vi "SA40144D.20210624 1D only.vi"() -> ()   [LabVIEW 2020]
uses:
  <vilib>/Analysis/baseanly.llb/Mean (DBL).vi
  <userlib>/_OpenG.lib/file/file.llb/Build Path - Traditional__ogtk.vi
  <userlib>/LevyLab/LV to ITX/Data/Data.lvclass
  <userlib>/LevyLab/XY Utilities/xy_utilities.lvlib
  <vilib>/Analysis/NI_AALBase.lvlib
panel:
  in  "Temps to keep (Lifespan)":i32=26
  out "Lifespan vs Temp (hrs)":cluster{i32[], dbl[]}[](graph)
  out "E_a":dbl[](array[numeric])
  out "Arrhenius":T1(graph)
  in  "Temps to keep (Arrhenius fit)":i32=26
  out "G2T vs t":T1(graph)
  out "G4T vs t":T1(graph)
  out "X5 - I-":T1(graph)
  out "X6 - dV":T1(graph)
  out "Temp vs t":T1(graph)
  out "G2T BG vs t":T1(graph)
  in  "Source Voltage":dbl=0.1
  in  "Init Temp":i32=275
  in  "Temp Step":i32=5
  in  "Final Temp":i32=360
  in  "Data File":path=path "G:/My Drive/ansom/Data/PPMS 2/SA40144D.20210624/00 - 1D only/SA40144D.20210624.000000.dat"
  in  "Trimming":i32=400
  in  "Update":bool
  in  "OK":bool
  out "error out":errorcluster
  in  "error in (no error)":errorcluster
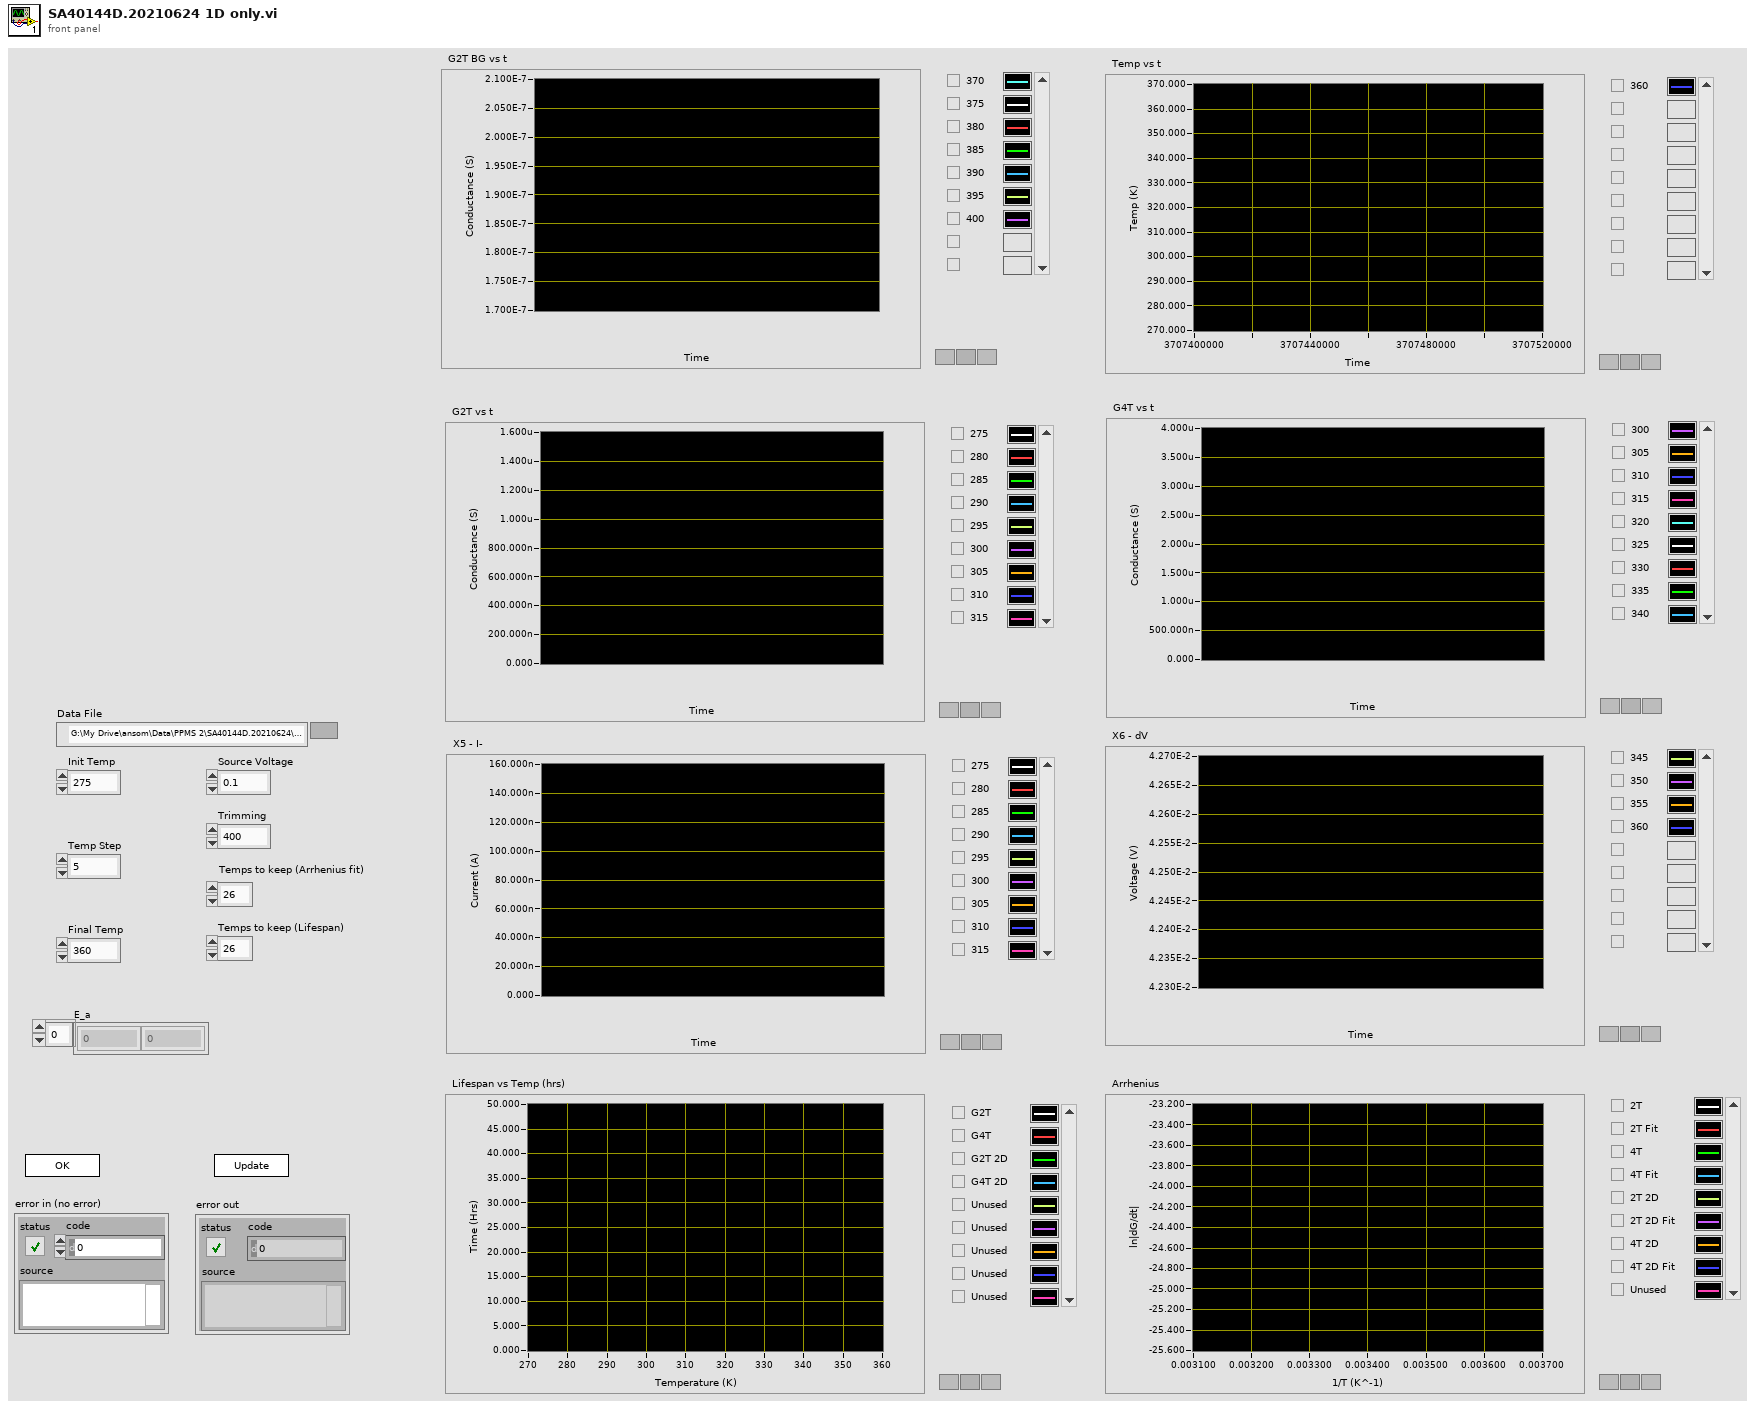
[diagram p1: front panel]
types:
  T1 = cluster{"Data":dbl[], "Best Exponential Fit":dbl[]}[]
  T2 = enum32{"Invalid", "Standard", "Closed", "Hidden", "Minimized", "Maximized"}
  T3 = enum32{"invalid app kind", "Development System", "Run Time System", "Student Edition", "Embedded LabVIEW", "Evaluation", "Custom"}
  T4 = cluster{"Core":cluster{"Current VI Reference":refnum<vi>, "Close Panel on Exit?":bool}, "G2T 1D":cluster{dbl[], dbl[]}[], "G4T 1D":cluster{dbl[], dbl[]}[], "X11":cluster{dbl[], dbl[]}[], "X15":cluster{dbl[], dbl[]}[], "Temp":cluster{dbl[], dbl[]}[], "G2T BG":cluster{dbl[], dbl[]}[], "Source Voltage":dbl, "Final Temp":i32, "Init Temp":i32, "Temp Step":i32, "Data File":path, "Trimming":i32}
  T5 = cluster{"Current VI Reference":refnum<vi>, "Close Panel on Exit?":bool}
  T6 = typedef "Data.lvclass/Dictionary--cluster.ctl" = cluster{"key":string, "value":variant}
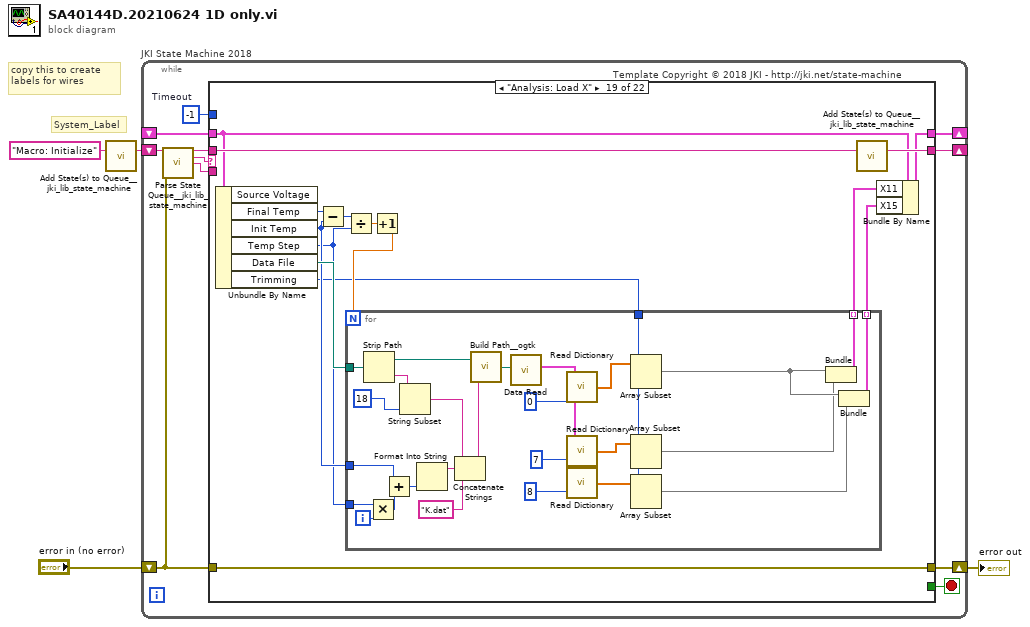
[diagram p0: block diagram]
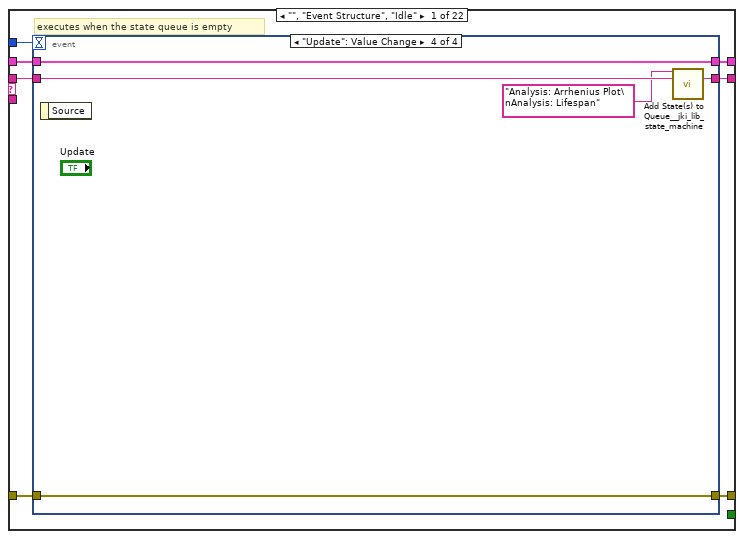
[diagram p2: hidden frame]
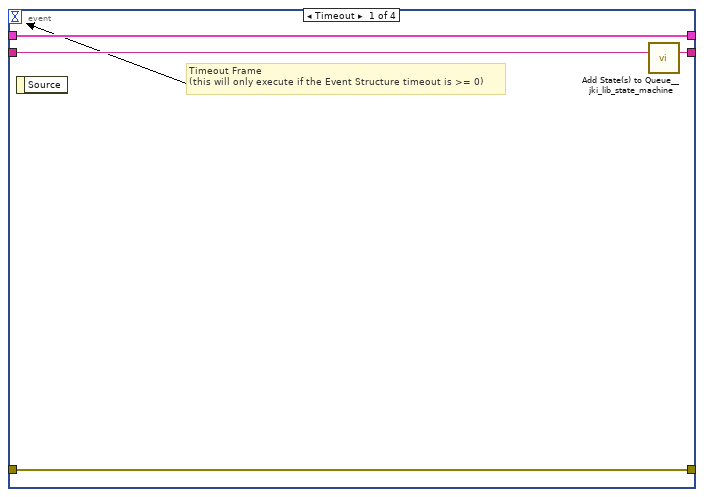
[diagram p3: hidden frame]
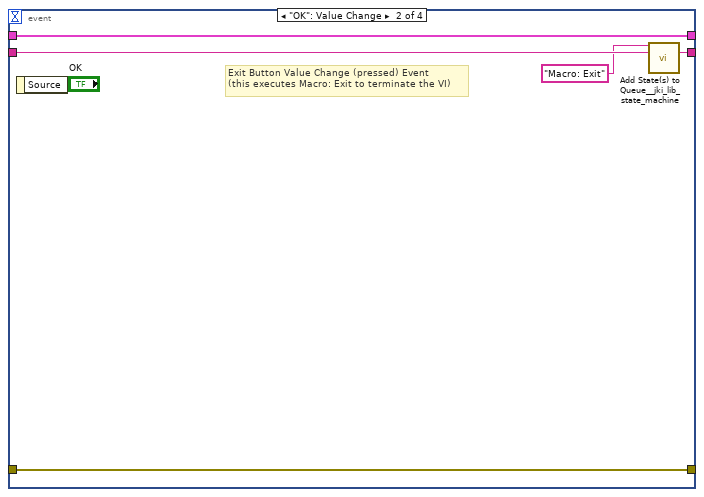
[diagram p4: hidden frame]
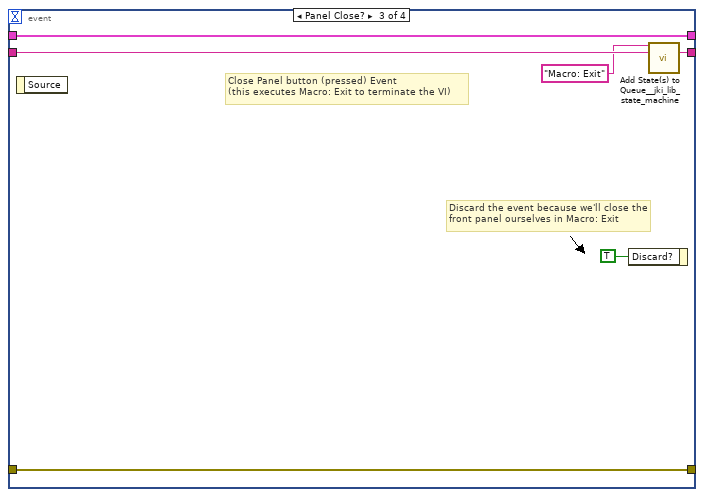
[diagram p5: hidden frame]
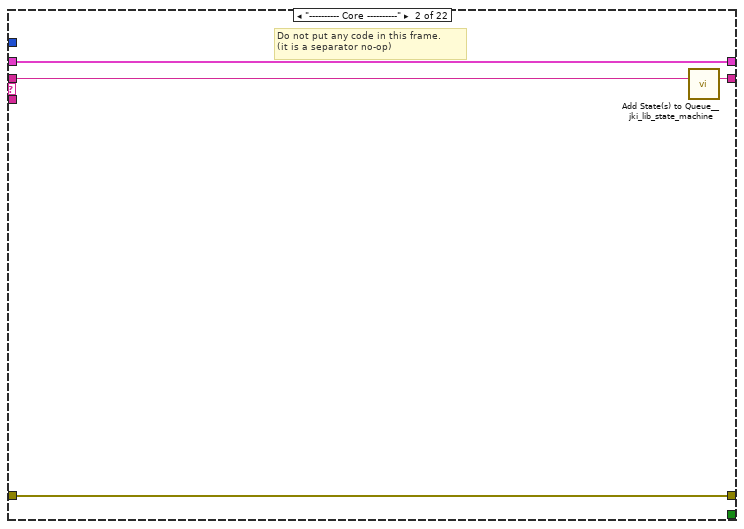
[diagram p6: hidden frame]
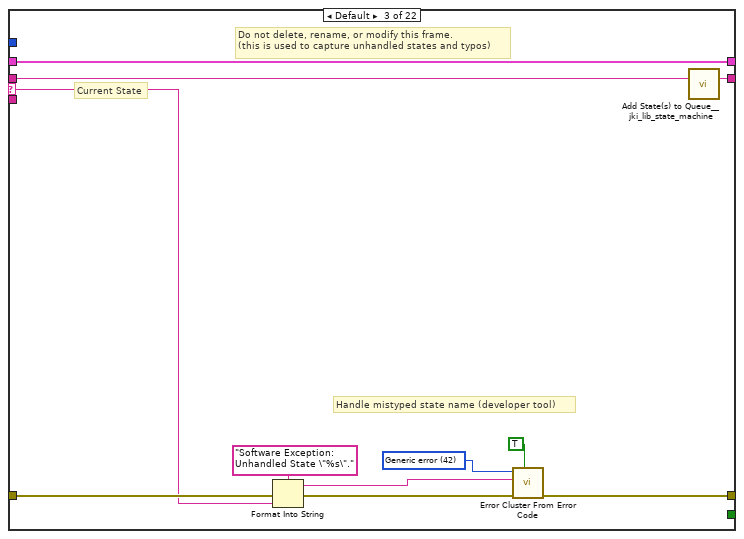
[diagram p7: hidden frame]
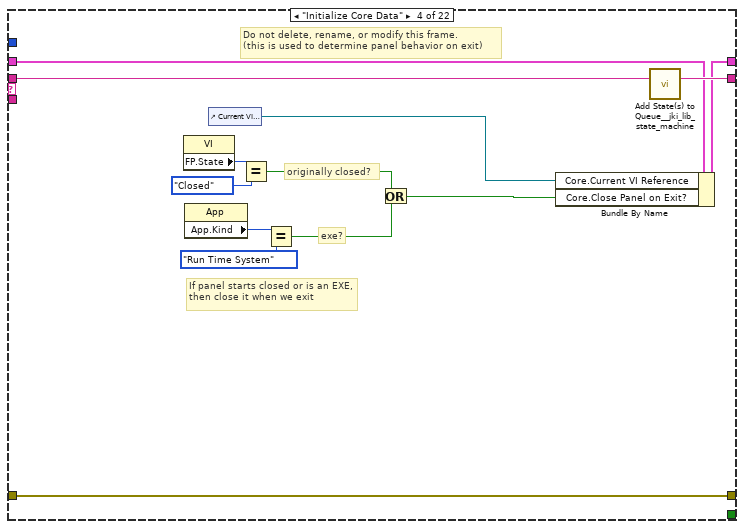
[diagram p8: hidden frame]
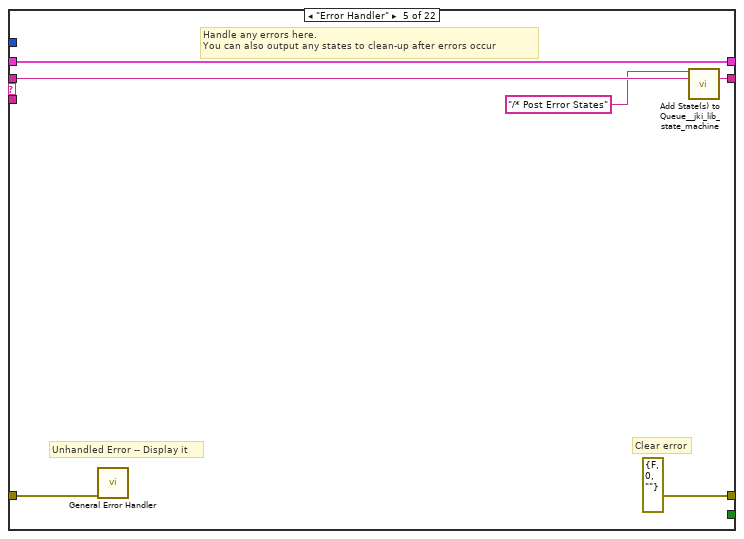
[diagram p9: hidden frame]
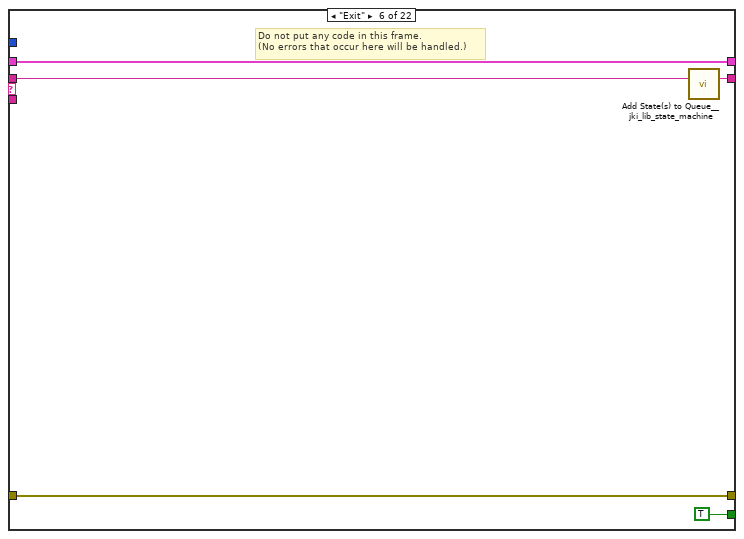
[diagram p10: hidden frame]
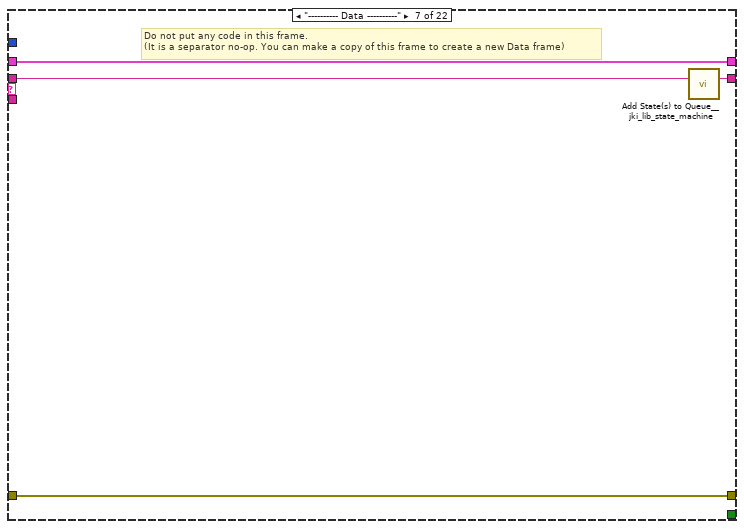
[diagram p11: hidden frame]
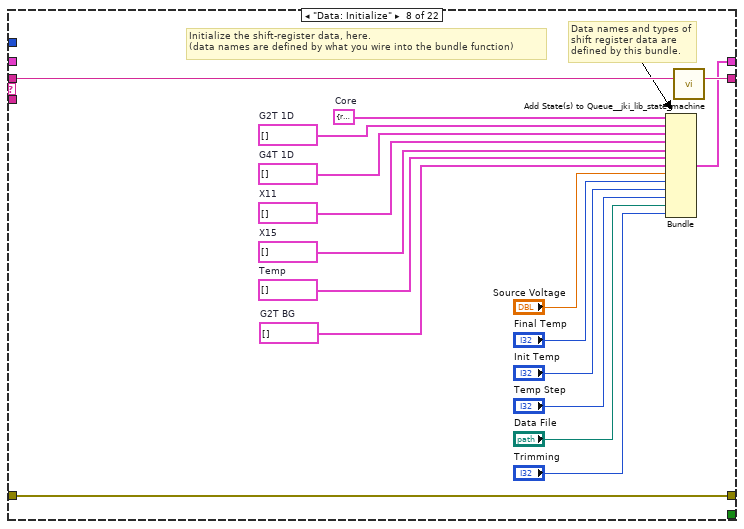
[diagram p12: hidden frame]
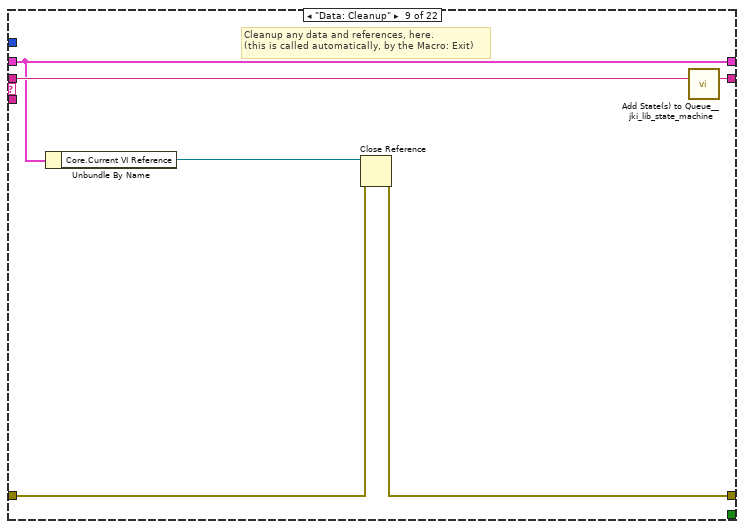
[diagram p13: hidden frame]
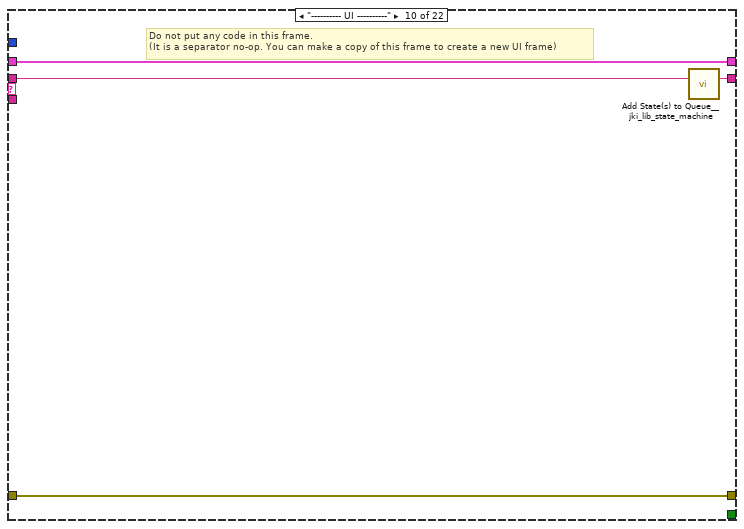
[diagram p14: hidden frame]
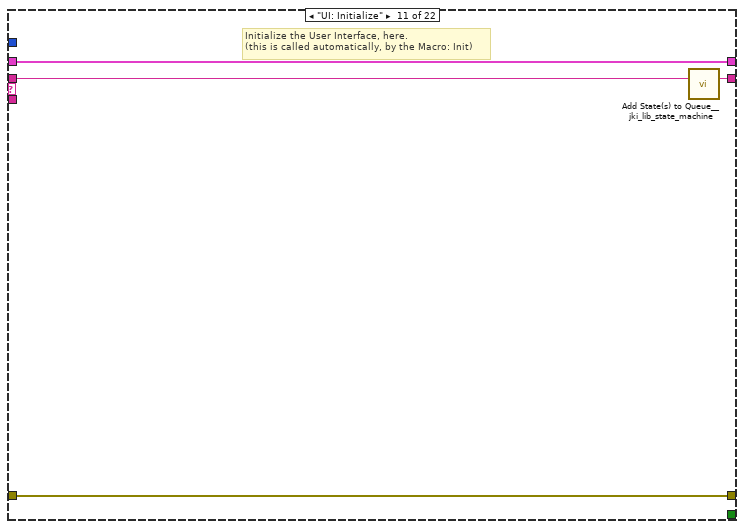
[diagram p15: hidden frame]
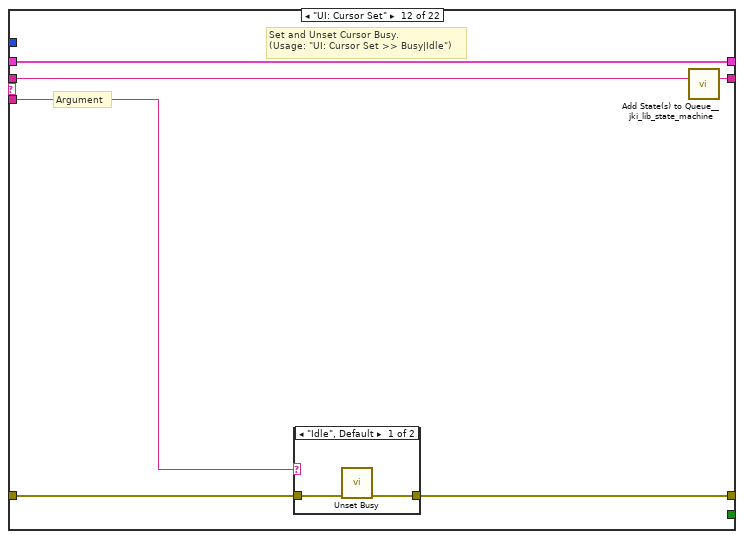
[diagram p16: hidden frame]
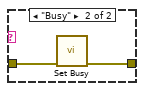
[diagram p17: hidden frame]
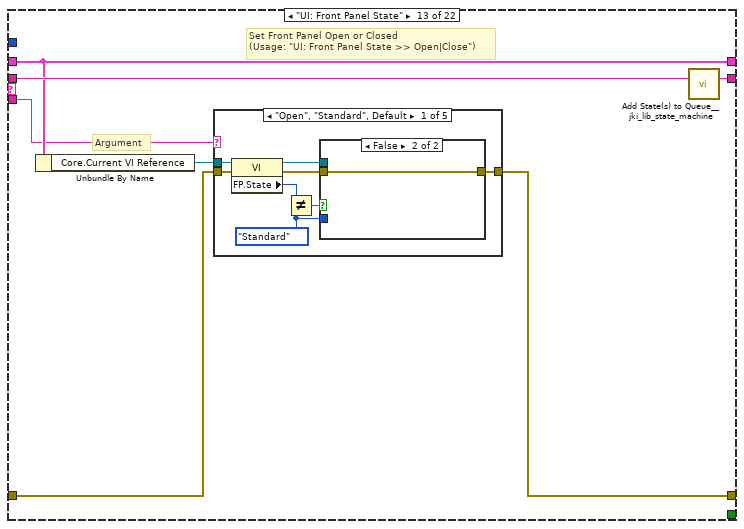
[diagram p18: hidden frame]
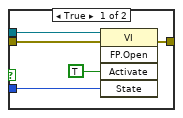
[diagram p19: hidden frame]
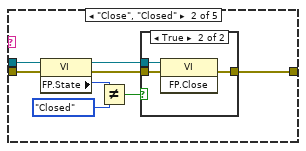
[diagram p20: hidden frame]
diagram:
  # "copy this to create labels for wires"
  # "System_Label"
  n1 = call <vilib>:"Add State(s) to Queue__jki_lib_state_machine.vi"("State(s) in (\"\")"="Macro: Initialize") -> ("States Out"=w4:string)  [unwired: 14 in]
  n2 = while "JKI State Machine 2018" {
    shift-right: [w8] -> _
    shift-left: _ -> [w7]
    shift-right: [w11] -> w1
    shift-left: "error in (no error)" -> [w5]
    shift-right: [w10] -> _
    shift-left: w4 -> [w12]
    stop <- w9 stop-if-true
    w6 = -1  # Timeout
    # "Template Copyright © 2018 JKI - http://jki.net/state-machine"
    n3 = call <vilib>:"Parse State Queue__jki_lib_state_machine.vi"("State Queue"=w12, "Error In (no error)"=w5) -> ("Remaining States"=w14:string, "Current State"=w15:string, "Arguments"=w13:string)  [unwired: 11 in]
    n4 = case shown="\"Analysis: Load X\"" w15 {
      selector: w15 -> [_ _ w47 _ _ _ _ _ _ _ _ _ _ _ _ _ _ _ _ _ _ _]
      tunnel: w14 -> [w22 w46 w51 w70 w76 w81 w85 w102 w108 w112 w116 w122 w133 w202 w207 w217 w221 w238 w289 w326 w358 w397]
      tunnel: w13 -> [_ _ _ _ _ _ _ _ _ _ _ w117 w127 _ _ _ _ _ _ _ _ _]
      tunnel: w7 -> [w20 w43 w49 w63 w73 w79 w82 _ w103 w109 w114 w120 w129 w199 w204 w214 w218 w232 w283 w323 w355 w383]
      tunnel: [w19 w44 w53 w67 errorcluster {"status"=FALSE, "code"=0, "source"=""} ("error out") w78 w83 w99 w104 w110 w113 w118 w130 w200 w205 w215 w219 w234 w285 w324 w356 w395] -> w11
      tunnel: w5 -> [w18 w44 w52 w67 w72 w78 w83 w99 w105 w110 w113 w119 w131 w200 w205 w215 w219 w234 w285 w324 w356 w395]
      tunnel: [w21 w45 w50 w69 w75 w80 w84 w101 w107 w111 w115 w121 w132 w201 w206 w216 w220 w237 w288 w325 w357 w396] -> w10
      tunnel: [_ _ _ _ _ TRUE _ _ _ _ _ _ _ _ _ _ _ _ _ _ _ _] -> w9
      tunnel: [w17 w43 w49 w68 w73 w79 w82 w100 w103 w109 w114 w120 w129 w199 w204 w214 w218 w233 w284 w323 w355 w383] -> w8
      tunnel: w6 -> [w16 _ _ _ _ _ _ _ _ _ _ _ _ _ _ _ _ _ _ _ _ _]
      frame "", "Event Structure", "Idle" {
        # "executes when the state queue is empty"
        n5 = event shown="[3] \"Update\": Value Change" {
          selector: _ -> [_ _ _ _]
          dyn-events: _ -> [_ _ _ _]
          timeout: w16 -> [_ _ _ _]
          tunnel: w22 -> [w26 w31 w37 w41]
          tunnel: [w25 w30 w36 w40] -> w21
          tunnel: w20 -> [w23 w28 w34 w42]
          tunnel: [w24 w29 w35 w38] -> w19
          tunnel: w18 -> [w24 w29 w35 w38]
          tunnel: [w23 w28 w34 w42] -> w17
          event Timeout {
            # "Timeout Frame\n(this will only execute if the Event Structure timeout is >= 0)"
            n6 = event-data() -> ()  [unwired: 1 in, 1 out]
            n7 = call <vilib>:"Add State(s) to Queue__jki_lib_state_machine.vi"("State(s) in (\"\")"=w26) -> ("States Out"=w25:string)  [unwired: 14 in]
          }
          event "OK": Value Change {
            # "Exit Button Value Change (pressed) Event\n(this executes Macro: Exit to terminate the VI)"
            n8 = event-data() -> ()  [unwired: 1 in, 1 out]
            n9 = call <vilib>:"Add State(s) to Queue__jki_lib_state_machine.vi"("State(s) in Front (\"\")"="Macro: Exit", "State(s) in (\"\")"=w31) -> ("States Out"=w30:string)  [unwired: 13 in]
          }
          event Panel Close? {
            # "Discard the event because we'll close the front panel ourselves in Macro: Exit"
            # "Close Panel button (pressed) Event\n(this executes Macro: Exit to terminate the VI)"
            n10 = event-data() -> ()  [unwired: 1 in, 1 out]
            n11 = event-data("Discard?"=TRUE) -> ()  [unwired: 1 in, 1 out]
            n12 = call <vilib>:"Add State(s) to Queue__jki_lib_state_machine.vi"("State(s) in Front (\"\")"="Macro: Exit", "State(s) in (\"\")"=w37) -> ("States Out"=w36:string)  [unwired: 13 in]
          }
          event "Update": Value Change {
            n13 = event-data() -> ()  [unwired: 1 in, 1 out]
            n14 = call <vilib>:"Add State(s) to Queue__jki_lib_state_machine.vi"("State(s) in Front (\"\")"="Analysis: Arrhenius Plot\nAnalysis: Lifespan" ("State(s) in Front (\"\")"), "State(s) in (\"\")"=w41) -> ("States Out"=w40:string)  [unwired: 13 in]
          }
        }
      }
      frame "---------- Core ----------" {
        # "Do not put any code in this frame.\n(it is a separator no-op)"
        n15 = call <vilib>:"Add State(s) to Queue__jki_lib_state_machine.vi"("State(s) in (\"\")"=w46) -> ("States Out"=w45:string)  [unwired: 14 in]
      }
      frame Default {
        w56 = 42 items=["No error", "Argument error", "Memory is full", "Out of zone", "End of file", "File already open", "Generic file I/O error", "File not found", "File permission error", "Disk is full", "Duplicate path", "Too many files open", "System feature not enabled", "Resource file not found", "Cannot add resource", "Resource not found", "Image not found", "Image memory error", "Pen does not exist", "Config type invalid", "Config token not found", "Config parse error", "Config memory error", "Bad external code format", "Bad external code offset", "External code not present", "Null window", "Destroy window error", "Null menu", "Print aborted", "Bad print record", "Print driver error", "Windows error during printing", "Memory error during printing", "Print dialog error", "Generic print error", "Invalid device refnum", "Device not found", "Device parameter error", "Device unit error", "Cannot open device", "Device call aborted", "Generic error", "Cancelled by user", "Object ID too low", "Object ID too high", "Object not in heap", "Unknown heap", "Unknown object (invalid DefProc)", "Unknown object (DefProc not in table)", "Message out of range", "Invalid (null) method", "Unknown message", "Manager call not supported", "Bad address", "Network operation in progress", "Network operation timed out", "Connection is busy", "Network attribute not supported", "Network error", "Address in use", "System out of memory", "Connection aborted", "Connection refused", "Not connected", "Already connected", "Connection closed", "Initialization error (interapplication manager)", "Bad occurrence", "Wait on unbound occurrence handler", "Occurrence queue overflow", "Datalog type conflict", "Unused", "Unrecognized type (interapplication manager)", "Memory corrupt", "Failed to make temporary DLL", "Old CIN version", "Drag socket not found", "Failed to load drop-object", "Failed to register OLE object", "Failed to release OLE object", "Format specifier type mismatch", "Unknown format specifier", "Too few format specifiers", "Too many format specifiers", "Scan failed", "Newer CIN version", "Error converting to variant", "Runtime menu error", "Password tampered", "Variant attribute not found", "Incompatible variant data type", "Event data is not available", "Event Store is not present", "Occurrence is not found", "Event Queue is not created", "Event info is not available", "Refnum passed is NULL", "Error retrieving Class GUID", "Error retrieving CoClass GUID", "Error retrieving TypeLib GUID.", "Bad built application magic bytes.", "Specific driver is different from the specific driver associated with the Logical Name.", "There is no session opened to the class driver.", "Max Error", "MAX - Error with config objects", "MAX - Error loading configuration", "MAX - Group not supported"]
        # "Current State"
        # "Do not delete, rename, or modify this frame.\n(this is used to capture unhandled states and typos)"
        # "Handle mistyped state name (developer tool)"
        n16 = Format Into String(format string="Software Exception: Unhandled State \"%s\"." ("message"), error in=w52, w47) -> (resulting string=w55:string, error out=w54:errorcluster)  [unwired: 1 in]
        n17 = call <vilib>:"Error Cluster From Error Code.vi"("show call chain? (False)"=TRUE, "error in (no error)"=w54, "error message (\"\")"=w55, "error code (0)"=w56) -> ("error out"=w53:errorcluster)  [unwired: 5 in]
        n18 = call <vilib>:"Add State(s) to Queue__jki_lib_state_machine.vi"("State(s) in (\"\")"=w51) -> ("States Out"=w50:string)  [unwired: 14 in]
      }
      frame "Initialize Core Data" {
        # "Do not delete, rename, or modify this frame.\n(this is used to determine panel behavior on exit)"
        # "originally closed?"
        # "exe?"
        # "If panel starts closed or is an EXE, then close it when we exit"
        n19 = property class="VI"() -> ("FP.State"=w60:T2)  [unwired: 2 in, 2 out]
        n20 = property class="App"() -> ("App.Kind"=w66:T3)  [unwired: 2 in, 2 out]
        n21 = control-ref of="Current VI Reference"() -> (w61:refnum<vi>)
        n22 = Equal?(x=w60, y=T2."Closed" ("Front Panel Window:State")) -> (x = y?=w58:bool)
        n23 = Equal?(x=w66, y=T3."Run Time System" ("Application:Kind")) -> (x = y?=w64:bool)
        n24 = Or(x=w58, y=w64) -> (x .or. y?=w62:bool)
        n25 = Bundle By Name(cluster=w63, "Core.Current VI Reference"=w61, "Core.Close Panel on Exit?"=w62) -> (w68:T4)
        n26 = call <vilib>:"Add State(s) to Queue__jki_lib_state_machine.vi"("State(s) in (\"\")"=w70) -> ("States Out"=w69:string)  [unwired: 14 in]
      }
      frame "Error Handler" {
        # "Unhandled Error -- Display it"
        # "Handle any errors here.\nYou can also output any states to clean-up after errors occur"
        # "Clear error"
        n27 = call <vilib>:"General Error Handler.vi"("error in (no error)"=w72) -> ()  [unwired: 10 in, 5 out]
        n28 = call <vilib>:"Add State(s) to Queue__jki_lib_state_machine.vi"("State(s) in Front (\"\")"="/* Post Error States", "State(s) in (\"\")"=w76) -> ("States Out"=w75:string)  [unwired: 13 in]
      }
      frame "Exit" {
        # "Do not put any code in this frame.\n(No errors that occur here will be handled.)"
        n29 = call <vilib>:"Add State(s) to Queue__jki_lib_state_machine.vi"("State(s) in (\"\")"=w81) -> ("States Out"=w80:string)  [unwired: 14 in]
      }
      frame "---------- Data ----------" {
        # "Do not put any code in this frame.\n(It is a separator no-op. You can make a copy of this frame to create a new Data frame)"
        n30 = call <vilib>:"Add State(s) to Queue__jki_lib_state_machine.vi"("State(s) in (\"\")"=w85) -> ("States Out"=w84:string)  [unwired: 14 in]
      }
      frame "Data: Initialize" {
        w86 = cluster{dbl[], dbl[]}[] []  # G2T BG
        w87 = cluster{dbl[], dbl[]}[] []  # Temp
        w96 = cluster{dbl[], dbl[]}[] []  # X15
        w95 = cluster{dbl[], dbl[]}[] []  # X11
        w94 = cluster{dbl[], dbl[]}[] []  # G4T 1D
        w93 = cluster{dbl[], dbl[]}[] []  # G2T 1D
        w98 = T5 {"Current VI Reference"=refnum, "Close Panel on Exit?"=FALSE}  # Core
        # "Data names and types of shift register data are defined by this bundle."
        # "Initialize the shift-register data, here.\n(data names are defined by what you wire into the bundle function)"
        n31 = Bundle("Core"=w98, "G2T 1D"=w93, "G4T 1D"=w94, "X11"=w95, "X15"=w96, "Temp"=w87, "G2T BG"=w86, "Source Voltage"="Source Voltage", "Final Temp"="Final Temp", "Init Temp"="Init Temp", "Temp Step"="Temp Step", "Data File"="Data File", "Trimming"="Trimming") -> (w100:T4)  [unwired: 1 in]
        n32 = call <vilib>:"Add State(s) to Queue__jki_lib_state_machine.vi"("State(s) in (\"\")"=w102) -> ("States Out"=w101:string)  [unwired: 14 in]
      }
      frame "Data: Cleanup" {
        # "Cleanup any data and references, here.\n(this is called automatically, by the Macro: Exit)"
        n33 = Unbundle By Name(w103) -> ("Core.Current VI Reference"=w106:refnum<vi>)
        n34 = Close Reference(reference=w106, error in (no error)=w105) -> (error out=w104:errorcluster)
        n35 = call <vilib>:"Add State(s) to Queue__jki_lib_state_machine.vi"("State(s) in (\"\")"=w108) -> ("States Out"=w107:string)  [unwired: 14 in]
      }
      frame "---------- UI ----------" {
        # "Do not put any code in this frame.\n(It is a separator no-op. You can make a copy of this frame to create a new UI frame)"
        n36 = call <vilib>:"Add State(s) to Queue__jki_lib_state_machine.vi"("State(s) in (\"\")"=w112) -> ("States Out"=w111:string)  [unwired: 14 in]
      }
      frame "UI: Initialize" {
        # "Initialize the User Interface, here.\n(this is called automatically, by the Macro: Init)"
        n37 = call <vilib>:"Add State(s) to Queue__jki_lib_state_machine.vi"("State(s) in (\"\")"=w116) -> ("States Out"=w115:string)  [unwired: 14 in]
      }
      frame "UI: Cursor Set" {
        # "Argument"
        # "Set and Unset Cursor Busy.\n(Usage: \"UI: Cursor Set >> Busy|Idle\")"
        n38 = case shown="\"Idle\", Default" w117 {
          tunnel: w119 -> [w124 w126]
          tunnel: [w123 w125] -> w118
          frame "Idle", Default {
            n39 = call <vilib>:"Unset Busy.vi"("error in (no error)"=w124) -> ("error out"=w123:errorcluster)  [unwired: 10 in]
          }
          frame "Busy" {
            n40 = call <vilib>:"Set Busy.vi"("error in (no error)"=w126) -> ("error out"=w125:errorcluster)  [unwired: 9 in, 1 out]
          }
        }
        n41 = call <vilib>:"Add State(s) to Queue__jki_lib_state_machine.vi"("State(s) in (\"\")"=w122) -> ("States Out"=w121:string)  [unwired: 14 in]
      }
      frame "UI: Front Panel State" {
        # "Argument"
        # "Set Front Panel Open or Closed\n(Usage: \"UI: Front Panel State >> Open|Close\")"
        n42 = Unbundle By Name(w129) -> ("Core.Current VI Reference"=w128:refnum<vi>)
        n43 = case shown="\"Open\", \"Standard\", Default" w127 {
          tunnel: w131 -> [w139 w154 w165 w178 w191]
          tunnel: [w141 w155 w167 w180 w193] -> w130
          tunnel: w128 -> [w140 w152 w166 w179 w192]
          frame "Open", "Standard", Default {
            w134 = T2."Standard" ("State")
            n44 = property class="VI"(reference=w140, error in=w139) -> (reference out=w137:refnum<vi>, error out=w138:errorcluster, "FP.State"=w136:T2)
            n45 = Not Equal?(x=w136, y=w134) -> (x != y?=w135:bool)
            n46 = case shown="False" w135 {
              tunnel: [w145 w147] -> w141
              tunnel: w138 -> [w144 w147]
              tunnel: w137 -> [w143 _]
              tunnel: w134 -> [w142 _]
              frame True {
                n47 = invoke class="VI" method="FP.Open"(reference=w143, error in=w144, "Activate"=TRUE, "State"=w142) -> (error out=w145:errorcluster)  [unwired: 1 in, 4 out]
              }
              frame False {
              }
            }
          }
          frame "Close", "Closed" {
            n48 = property class="VI"(reference=w152, error in=w154) -> (reference out=w151:refnum<vi>, error out=w153:errorcluster, "FP.State"=w149:T2)
            n49 = Not Equal?(x=w149, y=T2."Closed" ("Front Panel Window:State")) -> (x != y?=w148:bool)
            n50 = case shown="True" w148 {
              tunnel: [w156 w159] -> w155
              tunnel: w153 -> [w156 w158]
              tunnel: w151 -> [_ w157]
              frame False {
              }
              frame True {
                n51 = invoke class="VI" method="FP.Close"(reference=w157, error in=w158) -> (error out=w159:errorcluster)  [unwired: 1 in, 2 out]
              }
            }
          }
          frame "Hidden", "Hide" {
            w160 = T2."Hidden" ("State")
            n52 = property class="VI"(reference=w166, error in=w165) -> (reference out=w163:refnum<vi>, error out=w164:errorcluster, "FP.State"=w162:T2)
            n53 = Not Equal?(x=w162, y=w160) -> (x != y?=w161:bool)
            n54 = case shown="True" w161 {
              tunnel: [w171 w172] -> w167
              tunnel: w164 -> [w170 w172]
              tunnel: w163 -> [w169 _]
              tunnel: w160 -> [w168 _]
              frame True {
                n55 = invoke class="VI" method="FP.Open"(reference=w169, error in=w170, "State"=w168) -> (error out=w171:errorcluster)  [unwired: 2 in, 4 out]
              }
              frame False {
              }
            }
          }
          frame "Minimize", "Minimized" {
            w173 = T2."Minimized" ("State")
            n56 = property class="VI"(reference=w179, error in=w178) -> (reference out=w176:refnum<vi>, error out=w177:errorcluster, "FP.State"=w175:T2)
            n57 = Not Equal?(x=w175, y=w173) -> (x != y?=w174:bool)
            n58 = case shown="True" w174 {
              tunnel: [w184 w185] -> w180
              tunnel: w177 -> [w183 w185]
              tunnel: w176 -> [w182 _]
              tunnel: w173 -> [w181 _]
              frame True {
                n59 = invoke class="VI" method="FP.Open"(reference=w182, error in=w183, "State"=w181) -> (error out=w184:errorcluster)  [unwired: 2 in, 4 out]
              }
              frame False {
              }
            }
          }
          frame "Maximize", "Maximized" {
            w186 = T2."Maximized" ("State")
            n60 = property class="VI"(reference=w192, error in=w191) -> (reference out=w189:refnum<vi>, error out=w190:errorcluster, "FP.State"=w188:T2)
            n61 = Not Equal?(x=w188, y=w186) -> (x != y?=w187:bool)
            n62 = case shown="True" w187 {
              tunnel: [w197 w198] -> w193
              tunnel: w190 -> [w196 w198]
              tunnel: w189 -> [w195 _]
              tunnel: w186 -> [w194 _]
              frame True {
                n63 = invoke class="VI" method="FP.Open"(reference=w195, error in=w196, "State"=w194) -> (error out=w197:errorcluster)  [unwired: 2 in, 4 out]
              }
              frame False {
              }
            }
          }
        }
        n64 = call <vilib>:"Add State(s) to Queue__jki_lib_state_machine.vi"("State(s) in (\"\")"=w133) -> ("States Out"=w132:string)  [unwired: 14 in]
      }
      frame "---------- Macro ----------" {
        # "Do not put any code in this frame.\n(It is a separator no-op. You can make a copy of this frame to create a new Macro frame)"
        n65 = call <vilib>:"Add State(s) to Queue__jki_lib_state_machine.vi"("State(s) in (\"\")"=w202) -> ("States Out"=w201:string)  [unwired: 14 in]
      }
      frame "Macro: Initialize" {
        # "Initialization Macro\n(This is called once, when the VI starts)"
        n66 = call <vilib>:"Add State(s) to Queue__jki_lib_state_machine.vi"("State(s) in Front (\"\")"="Data: Initialize\nInitialize Core Data\nUI: Initialize\nUI: Front Panel State >> Open\nAnalysis: Load 1D\nAnalysis: Load X\nAnalysis: Plot G vs t\nAnalysis: Arrhenius Plot\nAnalysis: Lifespan", "State(s) in (\"\")"=w207) -> ("States Out"=w206:string)  [unwired: 13 in]
      }
      frame "Macro: Exit" {
        # "Exit Macro\n(This is called once, when the VI exits)"
        n67 = Unbundle By Name(w214) -> ("Core.Close Panel on Exit?"=w213:bool)
        n68 = Select(t="UI: Front Panel State >> Close", s=w213, f="") -> (s? t:f=w210:string)
        n69 = call <vilib>:"Add State(s) to Queue__jki_lib_state_machine.vi"("State(s) in (\"\")"=w210, "State(s) at Back (\"\")"="Data: Cleanup\nExit") -> ("States Out"=w208:string)  [unwired: 13 in]
        n70 = call <vilib>:"Add State(s) to Queue__jki_lib_state_machine.vi"("State(s) in Front (\"\")"=w208, "State(s) in (\"\")"=w217) -> ("States Out"=w216:string)  [unwired: 13 in]
      }
      frame "---------- Analysis ----------" {
        # "Template Separator\n(You can make a copy of, or modify, this frame)"
        n71 = call <vilib>:"Add State(s) to Queue__jki_lib_state_machine.vi"("State(s) in (\"\")"=w221) -> ("States Out"=w220:string)  [unwired: 14 in]
      }
      frame "Analysis: Load 1D" {
        n72 = Unbundle By Name(w232) -> ("Source Voltage"=w231:dbl, "Final Temp"=w228:i32, "Init Temp"=w225:i32, "Temp Step"=w224:i32, "Data File"=w226:path, "Trimming"=w223:i32)
        n73 = Subtract(x=w228, y=w225) -> (x-y=w235:i32)
        n74 = Divide(x=w235, y=w224) -> (x/y=w236:dbl)
        n75 = Increment(x=w236) -> (x+1=w227:dbl)
        n76 = for {
          N: w227 -> [_]
          tunnel: w231 -> [w244]
          tunnel: [w262] -> w230 mode=indexing
          tunnel: [w261] -> w229 mode=indexing
          tunnel: w226 -> [w260]
          tunnel: w225 -> [w259]
          tunnel: w224 -> [w258]
          tunnel: w223 -> [w257]
          tunnel: [w254] -> w222 mode=indexing
          i -> [w265]
          n77 = Strip Path(path=w260) -> (stripped path=w270:path, name=w269:string)
          n78 = Multiply(x=w258, y=w265) -> (x*y=w266:i32)
          n79 = Add(x=w259, y=w266) -> (x+y=w271:i32)
          n80 = String Subset(string=w269, length (rest)=18) -> (substring=w267:string)  [unwired: 1 in]
          n81 = Format Into String(w271) -> (resulting string=w273:string)  [unwired: 3 in, 1 out]
          n82 = Concatenate Strings(w267, w273, "K.dat" ("string")) -> (w272:string)
          n83 = call-poly <userlib>:"Build Path__ogtk.vi"("name or relative path"=w272, "base path"=w270) -> ("appended path"=w274:path)
          n84 = call <userlib>:"Data Read.vi"("path"=w274) -> ("Data (Dictionary)"=w253:T6[])  [unwired: 7 in, 3 out]
          n85 = call "Read Dictionary.vi"("Numeric"=0, "Dictionary In"=w253) -> ("data"=w249:dbl[])
          n86 = call "Read Dictionary.vi"("Numeric"=7 ("index"), "Dictionary In"=w253) -> ("data"=w245:dbl[])
          n87 = call "Read Dictionary.vi"("Numeric"=8, "Dictionary In"=w253) -> ("data"=w248:dbl[])
          n88 = call "Read Dictionary.vi"("Numeric"=1, "Dictionary In"=w253) -> ("data"=w247:dbl[])
          n89 = Array Subset(array=w249, index=w257) -> (w256:dbl[])  [unwired: 1 in]
          n90 = Array Subset(array=w245, index=w257) -> (w243:dbl[])  [unwired: 1 in]
          n91 = Array Subset(array=w248, index=w257) -> (w242:dbl[])  [unwired: 1 in]
          n92 = Divide(x=w243, y=w244) -> (x/y=w264:dbl[])
          n93 = Absolute Value(x=w264) -> (abs(x)=w241:dbl[])
          n94 = Array Subset(array=w247) -> (w255:dbl[])  [unwired: 2 in]
          n95 = Divide(x=w243, y=w242) -> (x/y=w239:dbl[])
          n96 = Bundle(w256, w241) -> (w262:cluster{dbl[], dbl[]})  [unwired: 1 in]
          n97 = Bundle(w256, w255) -> (w254:cluster{dbl[], dbl[]})  [unwired: 1 in]
          n98 = Absolute Value(x=w239) -> (abs(x)=w240:dbl[])
          n99 = Bundle(w256, w240) -> (w261:cluster{dbl[], dbl[]})  [unwired: 1 in]
        }
        n100 = call <vilib>:"Add State(s) to Queue__jki_lib_state_machine.vi"("State(s) in (\"\")"=w238) -> ("States Out"=w237:string)  [unwired: 14 in]
        n101 = Bundle By Name(cluster=w232, "G2T 1D"=w230, "G4T 1D"=w229, "Temp"=w222) -> (w233:T4)
      }
      frame "Analysis: Load X" {
        n102 = Unbundle By Name(w283) -> ("Final Temp"=w281:i32, "Init Temp"=w278:i32, "Temp Step"=w277:i32, "Data File"=w279:path, "Trimming"=w276:i32)  [unwired: 1 out]
        n103 = Subtract(x=w281, y=w278) -> (x-y=w286:i32)
        n104 = Divide(x=w286, y=w277) -> (x/y=w287:dbl)
        n105 = Increment(x=w287) -> (x+1=w280:dbl)
        n106 = for {
          N: w280 -> [_]
          tunnel: [w305] -> w275 mode=indexing
          tunnel: [w304] -> w282 mode=indexing
          tunnel: w279 -> [w303]
          tunnel: w278 -> [w302]
          tunnel: w277 -> [w301]
          tunnel: w276 -> [w300]
          i -> [w307]
          n107 = Strip Path(path=w303) -> (stripped path=w312:path, name=w311:string)
          n108 = Multiply(x=w301, y=w307) -> (x*y=w308:i32)
          n109 = Add(x=w302, y=w308) -> (x+y=w313:i32)
          n110 = String Subset(string=w311, length (rest)=18) -> (substring=w309:string)  [unwired: 1 in]
          n111 = Format Into String(w313) -> (resulting string=w315:string)  [unwired: 3 in, 1 out]
          n112 = Concatenate Strings(w309, w315, "K.dat" ("string")) -> (w314:string)
          n113 = call-poly <userlib>:"Build Path__ogtk.vi"("name or relative path"=w314, "base path"=w312) -> ("appended path"=w316:path)
          n114 = call <userlib>:"Data Read.vi"("path"=w316) -> ("Data (Dictionary)"=w298:T6[])  [unwired: 7 in, 3 out]
          n115 = call "Read Dictionary.vi"("Numeric"=0, "Dictionary In"=w298) -> ("data"=w295:dbl[])
          n116 = call "Read Dictionary.vi"("Numeric"=7 ("index"), "Dictionary In"=w298) -> ("data"=w292:dbl[])
          n117 = call "Read Dictionary.vi"("Numeric"=8, "Dictionary In"=w298) -> ("data"=w294:dbl[])
          n118 = Array Subset(array=w295, index=w300) -> (w299:dbl[])  [unwired: 1 in]
          n119 = Array Subset(array=w292, index=w300) -> (w290:dbl[])  [unwired: 1 in]
          n120 = Array Subset(array=w294, index=w300) -> (w291:dbl[])  [unwired: 1 in]
          n121 = Bundle(w299, w290) -> (w305:cluster{dbl[], dbl[]})  [unwired: 1 in]
          n122 = Bundle(w299, w291) -> (w304:cluster{dbl[], dbl[]})  [unwired: 1 in]
        }
        n123 = call <vilib>:"Add State(s) to Queue__jki_lib_state_machine.vi"("State(s) in (\"\")"=w289) -> ("States Out"=w288:string)  [unwired: 14 in]
        n124 = Bundle By Name(cluster=w283, "X11"=w275, "X15"=w282) -> (w284:T4)
      }
      frame "Analysis: Plot G vs t" {
        n125 = Unbundle By Name(w323) -> ("G2T 1D"=→"G2T vs t":cluster{dbl[], dbl[]}[], "G4T 1D"=→"G4T vs t":cluster{dbl[], dbl[]}[], "X11"=→"X5 - I-":cluster{dbl[], dbl[]}[], "X15"=→"X6 - dV":cluster{dbl[], dbl[]}[], "G2T BG"=→"G2T BG vs t":cluster{dbl[], dbl[]}[], "Temp"=→"Temp vs t":cluster{dbl[], dbl[]}[])
        n126 = call <vilib>:"Add State(s) to Queue__jki_lib_state_machine.vi"("State(s) in (\"\")"=w326) -> ("States Out"=w325:string)  [unwired: 14 in]
      }
      frame "Analysis: Arrhenius Plot" {
        n127 = Unbundle By Name(w355) -> ("G2T 1D"=w330:cluster{dbl[], dbl[]}[], "G4T 1D"=w329:cluster{dbl[], dbl[]}[], "Final Temp"=w352:i32, "Init Temp"=w350:i32, "Temp Step"=w349:i32)  [unwired: 1 out]
        n128 = Subtract(x=w352, y=w350) -> (x-y=w353:i32)
        n129 = Divide(x=w353, y=w349) -> (x/y=w354:dbl)
        n130 = Increment(x=w354) -> (x+1=w351:dbl)
        n131 = for {
          N: w351 -> [_]
          tunnel: w350 -> [w361]
          tunnel: w349 -> [w362]
          tunnel: [w359] -> w341 mode=indexing
          i -> [w363]
          n132 = Multiply(x=w362, y=w363) -> (x*y=w364:i32)
          n133 = Add(x=w361, y=w364) -> (x+y=w360:i32)
          n134 = Reciprocal(x=w360) -> (1/x=w359:dbl)
        }
        n135 = call-poly <userlib>:"Linear Fit.vi"("XY-data"=w330) -> ("slopes"=w327:dbl[])  [unwired: 4 in, 6 out]
        n136 = call-poly <userlib>:"Linear Fit.vi"("XY-data"=w329) -> ("slopes"=w328:dbl[])  [unwired: 4 in, 6 out]
        n137 = Absolute Value(x=w327) -> (abs(x)=w347:dbl[])
        n138 = Absolute Value(x=w328) -> (abs(x)=w348:dbl[])
        n139 = Natural Logarithm(1:w347) -> (0:w343:dbl[])
        n140 = Natural Logarithm(1:w348) -> (0:w342:dbl[])
        n141 = Array Subset(array=w343, length="Temps to keep (Arrhenius fit)") -> (w339:dbl[])  [unwired: 1 in]
        n142 = Array Subset(array=w342, length="Temps to keep (Arrhenius fit)") -> (w338:dbl[])  [unwired: 1 in]
        n143 = Array Subset(array=w341, length="Temps to keep (Arrhenius fit)") -> (w337:dbl[])  [unwired: 1 in]
        n144 = Bundle(w337, w339) -> (w345:cluster{dbl[], dbl[]})  [unwired: 1 in]
        n145 = Bundle(w337, w338) -> (w346:cluster{dbl[], dbl[]})  [unwired: 1 in]
        n146 = Build Array(w345, w346) -> (w334:cluster{dbl[], dbl[]}[])
        n147 = call-poly <userlib>:"Linear Fit.vi"("XY-data"=w334) -> ("Best Fits"=w333:cluster{"X-array":dbl[], "Y-array":dbl[]}[], "XY-data out"=w332:cluster{"X-array":dbl[], "Y-array":dbl[]}[], "slopes"=w331:dbl[])  [unwired: 4 in, 4 out]
        n148 = Multiply(x=w331, y=8.617333e-05) -> (x*y=→"E_a":dbl[])
        n149 = Interleave 1D Arrays(w332, w333) -> (→"Arrhenius":cluster{"X-array":dbl[], "Y-array":dbl[]}[])
        n150 = call <vilib>:"Add State(s) to Queue__jki_lib_state_machine.vi"("State(s) in (\"\")"=w358) -> ("States Out"=w357:string)  [unwired: 14 in]
      }
      frame "Analysis: Lifespan" {
        w369 = 3600
        # "Template Separator\n(You can make a copy of, or modify, this frame)"
        n151 = Unbundle By Name(w383) -> ("G2T 1D"=w394:cluster{dbl[], dbl[]}[], "G4T 1D"=w393:cluster{dbl[], dbl[]}[], "Final Temp"=w390:i32, "Init Temp"=w382:i32, "Temp Step"=w381:i32)  [unwired: 3 out]
        n152 = Subtract(x=w390, y=w382) -> (x-y=w391:i32)
        n153 = Divide(x=w391, y=w381) -> (x/y=w392:dbl)
        n154 = Increment(x=w392) -> (x+1=w380:dbl)
        n155 = for {
          N: w380 -> [_]
          tunnel: w382 -> [w406]
          tunnel: w381 -> [w405]
          tunnel: [w404] -> w379 mode=indexing
          i -> [w407]
          n156 = Multiply(x=w405, y=w407) -> (x*y=w408:i32)
          n157 = Add(x=w406, y=w408) -> (x+y=w404:i32)
        }
        n158 = call <userlib>:"Linear Fit (multiple).vi"("XY-data"=w394) -> ("XY-data out"=w376:cluster{"X-array":dbl[], "Y-array":dbl[]}[], "slopes"=w378:dbl[])  [unwired: 4 in, 5 out]
        n159 = call <userlib>:"Linear Fit (multiple).vi"("XY-data"=w393) -> ("XY-data out"=w375:cluster{"X-array":dbl[], "Y-array":dbl[]}[], "slopes"=w377:dbl[])  [unwired: 4 in, 5 out]
        n160 = for {
          tunnel: w376 -> [w402] mode=indexing
          tunnel: w375 -> [w403] mode=indexing
          tunnel: [w399] -> w374 mode=indexing
          tunnel: [w398] -> w373 mode=indexing
          n161 = Unbundle(w402) -> ("Y-array"=w400:dbl[])  [unwired: 1 out]
          n162 = Unbundle(w403) -> ("Y-array"=w401:dbl[])  [unwired: 1 out]
          n163 = call-poly <vilib>:"Mean.vi"("X"=w401) -> ("mean"=w398:dbl)  [unwired: 1 out]
          n164 = call-poly <vilib>:"Mean.vi"("X"=w400) -> ("mean"=w399:dbl)  [unwired: 1 out]
        }
        n165 = Divide(x=w374, y=w378) -> (x/y=w371:dbl[])
        n166 = Divide(x=w373, y=w377) -> (x/y=w370:dbl[])
        n167 = Divide(x=w371, y=w369) -> (x/y=w367:dbl[])
        n168 = Divide(x=w370, y=w369) -> (x/y=w368:dbl[])
        n169 = Array Subset(array=w367, length="Temps to keep (Lifespan)") -> (w386:dbl[])  [unwired: 1 in]
        n170 = Array Subset(array=w368, length="Temps to keep (Lifespan)") -> (w385:dbl[])  [unwired: 1 in]
        n171 = Array Subset(array=w379, length="Temps to keep (Lifespan)") -> (w384:i32[])  [unwired: 1 in]
        n172 = Absolute Value(x=w386) -> (abs(x)=w365:dbl[])
        n173 = Absolute Value(x=w385) -> (abs(x)=w366:dbl[])
        n174 = Bundle(w384, w365) -> (w388:cluster{i32[], dbl[]})  [unwired: 1 in]
        n175 = Bundle(w384, w366) -> (w389:cluster{i32[], dbl[]})  [unwired: 1 in]
        n176 = Build Array(w388, w389) -> (→"Lifespan vs Temp (hrs)":cluster{i32[], dbl[]}[])
        n177 = call <vilib>:"Add State(s) to Queue__jki_lib_state_machine.vi"("State(s) in (\"\")"=w397) -> ("States Out"=w396:string)  [unwired: 14 in]
      }
    }
  }
  "error out" <- w1
